vi "testingdigitalbus.vi"() -> ()   [LabVIEW 2015]
uses:
  <vilib>/myRIO/Instrument Drivers/Onboard IO/PWM/typedefs/PWM Reference.ctl
  <vilib>/myRIO/Common/Instrument Driver Framework/Utilities/typedefs/myRIO Generic Hardware Reference.ctl
  <vilib>/myRIO/Common/Instrument Driver Framework/Utilities/typedefs/Hardware Version Enum.ctl
  <vilib>/myRIO/Common/Instrument Driver Framework/Utilities/typedefs/myRIO v1.0 Reference.ctl
  <vilib>/myRIO/Common/Instrument Driver Framework/Utilities/typedefs/Generic FPGA Reference.ctl
  <vilib>/myRIO/Common/Instrument Driver Framework/myRIO v1.0/PWM/typedefs/PWM Channels Enum.ctl
  <vilib>/myRIO/Instrument Drivers/Onboard IO/PWM/typedefs/PWM Configuration.ctl
  <vilib>/userdefined/High Color/nirio_resource_hc.ctl
  <vilib>/myRIO/Common/Instrument Driver Framework/myRIO v1.0/PWM/vis/myRIO v1.1 Open PWM.vi
  <vilib>/myRIO/Common/Instrument Driver Framework/Utilities/vis/Validate Channels.vi
  <vilib>/myRIO/Common/Instrument Driver Framework/myRIO v1.0/PWM/vis/myRIO v1.0 Reserve PWM.vi
  <vilib>/myRIO/Common/Instrument Driver Framework/myRIO v1.0/PWM/vis/myRIO v1.0 Close PWM.vi
  <vilib>/myRIO/Common/Instrument Driver Framework/myRIO v1.0/PWM/vis/myRIO v1.0 Build MUX Configuration PWM.vi
  <vilib>/myRIO/Common/Instrument Driver Framework/myRIO v1.0/Resource Manager/vis/myRIO v1.0 Reserve Channel List.vi
  <vilib>/myRIO/Common/Instrument Driver Framework/myRIO v1.0/PWM/vis/myRIO v1.0 Unreserve PWM.vi
  <vilib>/myRIO/Common/Instrument Driver Framework/myRIO v1.0/Resource Manager/vis/myRIO v1.0 Create Configuration List.vi
  <vilib>/myRIO/Common/Instrument Driver Framework/myRIO v1.0/Resource Manager/vis/myRIO v1.0 Reserve Channel.vi
  <vilib>/myRIO/Common/Instrument Driver Framework/myRIO v1.0/Resource Manager/vis/myRIO v1.0 Unreserve Channel.vi
  <vilib>/myRIO/Common/Instrument Driver Framework/myRIO v1.0/Resource Manager/vis/myRIO v1.0 Unreserve Channel List.vi
  <vilib>/myRIO/Common/Instrument Driver Framework/myRIO v1.0/Resource Manager/vis/myRIO v1.0 Build Mutex Name.vi
  <vilib>/Utility/VariantDataType/GetNumericInfo.vi
  <vilib>/Utility/error.llb/Error Cluster From Error Code.vi
  <vilib>/myRIO/Common/Instrument Driver Framework/myRIO v1.0/myRIO v1.1 Open.vi
  <vilib>/myRIO/Common/Instrument Driver Framework/Utilities/vis/IO Manager.vi
  <vilib>/myRIO/Common/Instrument Driver Framework/Utilities/vis/Configuration Manager.vi
  <vilib>/myRIO/Common/Instrument Driver Framework/myRIO v1.0/Resource Manager/vis/myRIO v1.0 Configure IO.vi
  <vilib>/myRIO/Common/Instrument Driver Framework/myRIO v1.0/myRIO v1.0 Close.vi
  <vilib>/myRIO/Common/Instrument Driver Framework/myRIO v1.0/PWM/vis/myRIO v1.0 Write PWM.vi
  <vilib>/myRIO/Common/Instrument Driver Framework/myRIO v1.0/PWM/vis/myRIO v1.0 Shutdown PWM.vi
  <vilib>/FPGAPlugInAG/myRIO-1900/niLvFpga_Open_myRIO-1900.vi
  <vilib>/rvi/interface/common/dynamic/niFpgaDynamicAddResources.vi
  <vilib>/rvi/errors/niLvFpgaAdjustHostInterfaceError.vi
  <vilib>/FPGAPlugInAG/Dynamic/niLvFpga_Close_Dynamic.vi
  <vilib>/myRIO/Instrument Drivers/Onboard IO/PWM/vis/myRIO PWM Open.xnode
  <vilib>/rvi/interface/nirviOpenFPGA/nirviOpenFPGA.xnode
  FPGA Bitfiles/Milestone4_FPGATarget_FPGAReadSonars_MhsUmP2nS8s.lvbitx
  physical_robot/FPGA Read Sonars.vi
  <vilib>/rvi/interface/nirviReadWriteControl/nirviReadWriteControl.xnode
  <vilib>/rvi/interface/nirviCloseFPGA/nirviCloseFPGA.xnode
  NiFpgaLv.dll
  <vilib>/rvi/interface/Simulation/niFpgaSimulationCallBeginRW.vi
  <vilib>/myRIO/Instrument Drivers/Onboard IO/PWM/PWM.lvlib
panel:
  out "Time Per Loop":dbl
  out "Total Time Taken":u32
  out "Time After":u32
  out "TIme before":u32
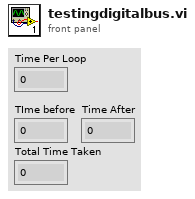
[diagram p1: front panel]
types:
  T1 = typedef "nirio_resource_hc.ctl" = tag
  T2 = typedef "Hardware Version Enum.ctl" = enum16{"Unknown", "myRIO-1900", "myRIO-1950", "roboRIO"}
  T3 = typedef "PWM.lvlib/PWM Reference.ctl" = cluster{"myRIO Reference":T4, "PWM Channels Enum":T7, "PWM Configuration":T8}
  T4 = typedef "myRIO Generic Hardware Reference.ctl" = cluster{"myRIO Model":T2, "myRIO Hardware Reference":T5}
  T5 = typedef "myRIO v1.0 Reference.ctl" = cluster{"Generic FPGA Reference":T6, "Allow multiple opens":bool}
  T6 = typedef "Generic FPGA Reference.ctl" = refnum<k20>
  T7 = typedef "PWM Channels Enum.ctl" = enum16{"Not Connected", "C/PWM0", "C/PWM1", "A/PWM0", "A/PWM1", "A/PWM2", "B/PWM0", "B/PWM1", "B/PWM2", "PWM/PWM0", "PWM/PWM1", "PWM/PWM2", "PWM/PWM3", "PWM/PWM4", "PWM/PWM5", "PWM/PWM6", "PWM/PWM7", "PWM/PWM8", "PWM/PWM9"}
  T8 = typedef "PWM.lvlib/PWM Configuration.ctl" = cluster{"Frequency":dbl, "Duty Cycle":dbl}
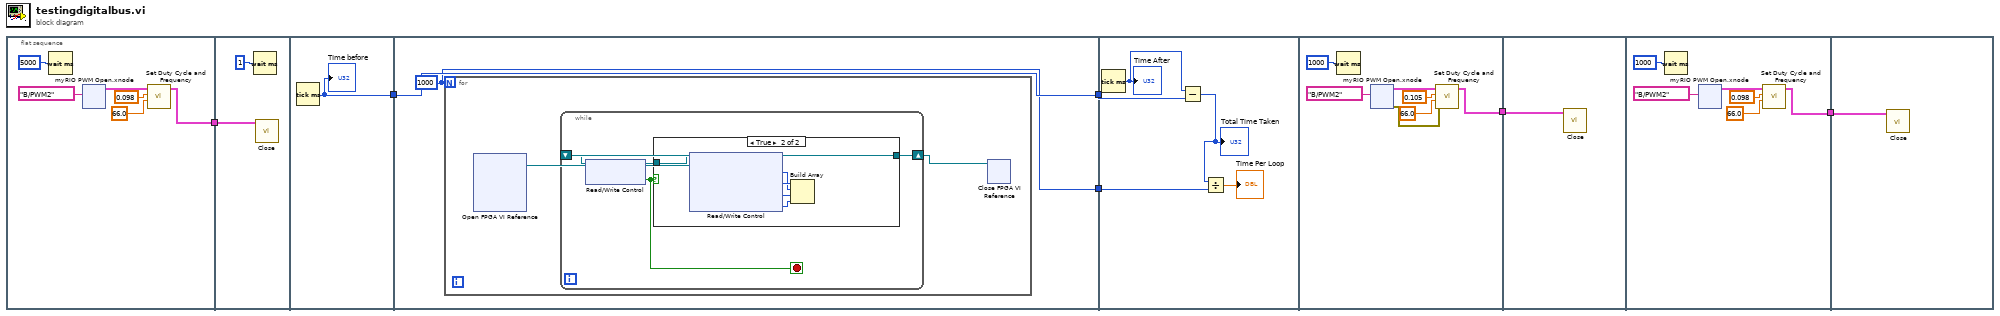
[diagram p0: block diagram]
diagram:
  n1 = flat-sequence {
    tunnel: [w7] -> w4
    tunnel: w4 -> [w29]
    tunnel: [w31] -> w6
    tunnel: w6 -> [w33]
    tunnel: [w33] -> w5
    tunnel: [w32] -> w1
    tunnel: w5 -> [w50]
    tunnel: w1 -> [w48]
    tunnel: [w52] -> w3
    tunnel: w3 -> [w75]
    tunnel: [w76] -> w2
    tunnel: w2 -> [w98]
    frame #0 {
      n2 = Wait (ms)(milliseconds to wait=u32 5000) -> ()  [unwired: 1 out]
      n3 = xnode "myRIO PWM Open.xnode"("Channel Name"=tag "B/PWM2") -> ("PWM Ref Out"=w11:T3)  [unwired: 2 in, 1 out]
      n4 = call <vilib>:"Set Duty Cycle and Frequency.vi"("Frequency [Hz]"=66.0, "Duty Cycle"=0.098, "PWM Ref In"=w11) -> ("PWM Ref Out"=w7:T3)  [unwired: 6 in, 1 out]
    }
    frame #1 {
      n5 = Wait (ms)(milliseconds to wait=u32 1) -> ()  [unwired: 1 out]
      n6 = call <vilib>:"Close.vi"("PWM Ref In"=w29) -> ()  [unwired: 10 in, 1 out]
    }
    frame #2 {
      n7 = Tick Count (ms)() -> (millisecond timer value=w31:u32)
      "TIme before" <- w31
    }
    frame #3 {
      w32 = 1000
      n8 = for {
        N: w32 -> [_]
        n9 = xnode "Open FPGA VI Reference"() -> ("FPGA VI Reference Out"=w35:refnum<k20>)  [unwired: 2 in, 1 out]
        n10 = while {
          shift-right: [w37] -> w34
          shift-left: w35 -> [w39]
          stop <- w36 stop-if-true
          n11 = xnode "Read/Write Control"("FPGA VI Reference In"=w39) -> ("FPGA VI Reference Out"=w38:refnum<k20>, "Read Ready"=w36:bool)  [unwired: 1 in, 1 out]
          n12 = case shown="True" w36 {
            tunnel: w38 -> [w40 w46]
            tunnel: [w40 w45] -> w37
            frame False {
            }
            frame True {
              n13 = xnode "Read/Write Control"("FPGA VI Reference In"=w46) -> ("FPGA VI Reference Out"=w45:refnum<k20>, "Time of Flight Front"=w44:u32, "Time of Flight Right"=w43:u32, "Time of Flight Back"=w42:u32, "Time of Flight Left"=w41:u32)  [unwired: 1 in, 1 out]
              n14 = Build Array(w44, w43, w42, w41) -> ()  [unwired: 1 out]
            }
          }
        }
        n15 = xnode "Close FPGA VI Reference"("FPGA VI Reference In"=w34) -> ()  [unwired: 1 in, 1 out]
      }
    }
    frame #4 {
      n16 = Tick Count (ms)() -> (millisecond timer value=w51:u32)
      "Time After" <- w51
      n17 = Subtract(x=w51, y=w50) -> (x-y=w49:u32)
      "Total Time Taken" <- w49
      n18 = Divide(x=w49, y=w48) -> (x/y=→"Time Per Loop":dbl)
    }
    frame #5 {
      n19 = Wait (ms)(milliseconds to wait=u32 1000) -> ()  [unwired: 1 out]
      n20 = xnode "myRIO PWM Open.xnode"("Channel Name"=tag "B/PWM2") -> ("error out"=w53:errorcluster, "PWM Ref Out"=w57:T3)  [unwired: 2 in]
      n21 = call <vilib>:"Set Duty Cycle and Frequency.vi"("error in (no error)"=w53, "Frequency [Hz]"=66.0, "Duty Cycle"=0.105, "PWM Ref In"=w57) -> ("PWM Ref Out"=w52:T3)  [unwired: 5 in, 1 out]
    }
    frame #6 {
      n22 = call <vilib>:"Close.vi"("PWM Ref In"=w75) -> ()  [unwired: 10 in, 1 out]
    }
    frame #7 {
      n23 = Wait (ms)(milliseconds to wait=u32 1000) -> ()  [unwired: 1 out]
      n24 = xnode "myRIO PWM Open.xnode"("Channel Name"=tag "B/PWM2") -> ("PWM Ref Out"=w80:T3)  [unwired: 2 in, 1 out]
      n25 = call <vilib>:"Set Duty Cycle and Frequency.vi"("Frequency [Hz]"=66.0, "Duty Cycle"=0.098, "PWM Ref In"=w80) -> ("PWM Ref Out"=w76:T3)  [unwired: 6 in, 1 out]
    }
    frame #8 {
      n26 = call <vilib>:"Close.vi"("PWM Ref In"=w98) -> ()  [unwired: 10 in, 1 out]
    }
  }
